vi "PushPullMachine.vi"() -> ()   [LabVIEW 2019]
doc: "Push-Pull device:\nCCD data queued so it can be saved and plotted, while it can go ahead with changing fields and so on.\nNotification is for when conditions are ready for a new shot."
panel:
  out "# waiting":i32
  out "latest notification":string
  out "Shift# 2":dbl
  out "Shift#":dbl
  out "notification 3":string="53 got Queue"
  out "notification 2":string="53 got Queue"
  in  "NotifierLoopDelay":u32=500
  in  "Queue Delay":u32=5000
  out "#passed":i32(graph)=17
  out "notification":string="53 got Queue"
  out "Queued number":i32=53
  in  "Pull back with Notifier":bool
  in  "Push to Queue":bool
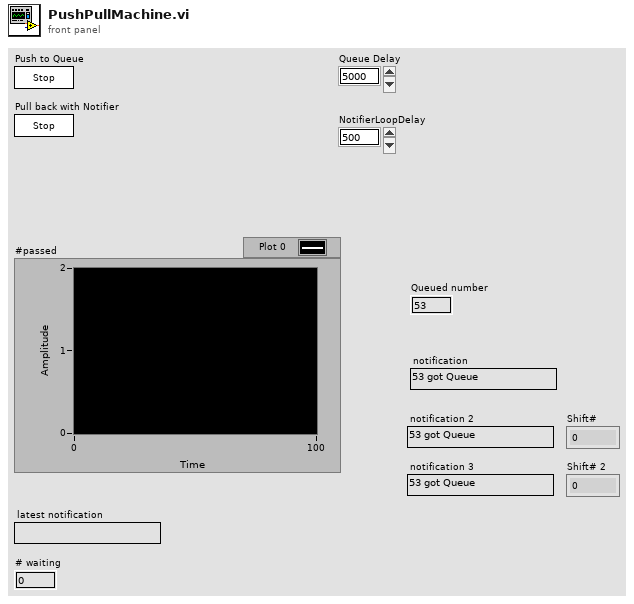
[diagram p1: front panel]
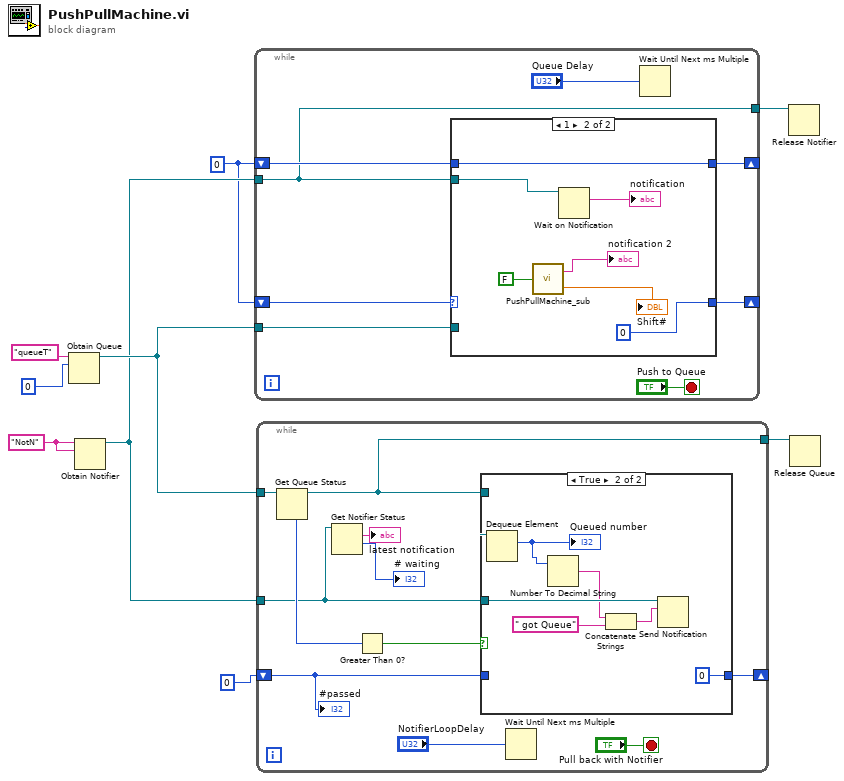
[diagram p0: block diagram]
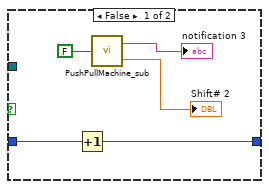
[diagram p2: hidden frame]
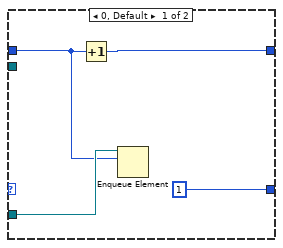
[diagram p3: hidden frame]
diagram:
  w6 = "NotN" ("name (unnamed)")
  w1 = 0
  n1 = Obtain Queue(name (unnamed)="queueT", element data type=0) -> (queue out=w7:refnum<queue>)  [unwired: 3 in, 2 out]
  n2 = Obtain Notifier(name (unnamed)=w6, notification data type=w6) -> (notifier out=w5:refnum<notifier>)  [unwired: 2 in, 2 out]
  n3 = while {
    shift-right: [w16] -> _
    shift-left: w1 -> [w17]
    shift-right: [w13] -> _
    shift-left: w1 -> [w14]
    tunnel: w7 -> [w12]
    tunnel: w5 -> [w10]
    tunnel: [w10] -> w2
    stop <- "Push to Queue" stop-if-true
    n4 = case shown="1" w17 {
      tunnel: [1 0] -> w16
      tunnel: w14 -> [w19 w26]
      tunnel: [w21 w26] -> w13
      tunnel: w12 -> [w20 _]
      tunnel: w10 -> [_ w27]
      frame 0, Default {
        n5 = Increment(x=w19) -> (x+1=w21:i32)
        n6 = Enqueue Element(queue=w20, element=w19) -> ()  [unwired: 2 in, 3 out]
      }
      frame 1 {
        n7 = call "PushPullMachine_sub.vi"("Notify?"=FALSE) -> ("notification"=→"notification 2":string, "Shift#"=→"Shift#":dbl)
        n8 = Wait on Notification(notifier=w27) -> (notification=→"notification":string)  [unwired: 3 in, 3 out]
      }
    }
    n9 = Wait Until Next ms Multiple(millisecond multiple="Queue Delay") -> ()  [unwired: 1 out]
  }
  n10 = while {
    shift-right: [w39] -> _
    shift-left: 0 -> [w34]
    tunnel: w7 -> [w37]
    tunnel: w5 -> [w29]
    tunnel: [w33] -> w3
    stop <- "Pull back with Notifier" stop-if-true
    n11 = Get Queue Status(queue=w37) -> (queue out=w33:refnum<queue>, # elements in queue=w36:i32)  [unwired: 2 in, 6 out]
    n12 = Get Notifier Status(notifier=w29) -> (current notification=→"latest notification":string, # waiting=→"# waiting":i32)  [unwired: 1 in, 3 out]
    n13 = Greater Than 0?(x=w36) -> (x > 0?=w35:bool)
    n14 = case shown="True" w35 {
      tunnel: [w43 0] -> w39
      tunnel: w33 -> [_ w51]
      tunnel: w29 -> [_ w50]
      tunnel: w34 -> [w44 _]
      frame False {
        n15 = Increment(x=w44) -> (x+1=w43:i32)
        n16 = call "PushPullMachine_sub.vi"("Notify?"=FALSE) -> ("notification"=→"notification 3":string, "Shift#"=→"Shift# 2":dbl)
      }
      frame True {
        n17 = Dequeue Element(queue=w51) -> (element=w49:i32)  [unwired: 2 in, 3 out]
        "Queued number" <- w49
        n18 = Number To Decimal String(number=w49) -> (decimal integer string=w48:string)  [unwired: 1 in]
        n19 = Concatenate Strings(w48, " got Queue" ("notification")) -> (w46:string)
        n20 = Send Notification(notification=w46, notifier=w50) -> ()  [unwired: 1 in, 2 out]
      }
    }
    n21 = Wait Until Next ms Multiple(millisecond multiple="NotifierLoopDelay") -> ()  [unwired: 1 out]
    "#passed" <- w34
  }
  n22 = Release Notifier(notifier=w2) -> ()  [unwired: 2 in, 3 out]
  n23 = Release Queue(queue=w3) -> ()  [unwired: 2 in, 3 out]
